vi "start.vi"(8 "error in (no error)":errorcluster, 10 "model":refnum<class "Model.lvclass">, 11 "StandbyState in":refnum<class "StandbyState.lvclass">) -> (0 "error out":errorcluster, 2 "model 2":refnum<class "Model.lvclass">, 3 "StandbyState out":refnum<class "StandbyState.lvclass">)   [LabVIEW 2013, in "StandbyState.lvclass"]
uses:
  StandbyState.lvclass
  Model/Model/Model.lvclass
  Typedefs/StateSelector.ctl
  Typedefs/AITDTTypedefs.lvlib
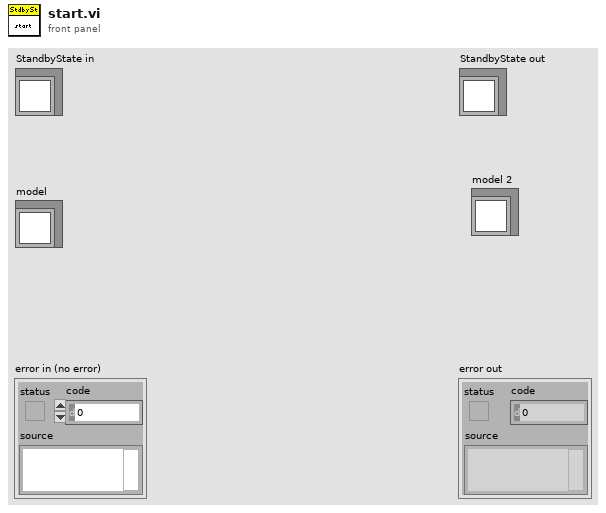
[diagram p1: front panel]
types:
  T1 = typedef "AITDTTypedefs.lvlib/StateSelector.ctl" = enum16{"AwaitingSetpointAcknowledgmentState", "EndingCycleState", "FaultState", "OffState", "PausingState", "RequestingNewSetpointState", "SamplingState", "SettlingState", "SoakingState", "StabilizingState", "StandbyState", "StoppedState", "TransitioningTemperatureState"}
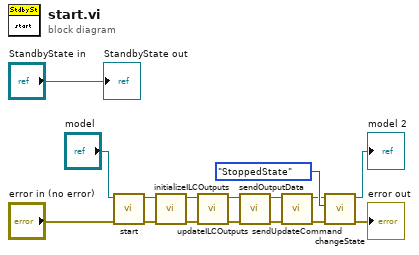
[diagram p0: block diagram]
diagram:
  n1 = call "start.vi"("error in (no error)"="error in (no error)", "Model in"="model") -> ("error out"=w9:errorcluster, "Model out"=w10:refnum<class "Model.lvclass">)  [unwired: 8 in]
  n2 = call "initializeILCOutputs.vi"("error in (no error)"=w9, "Model in"=w10) -> ("error out"=w1:errorcluster, "Model out"=w2:refnum<class "Model.lvclass">)  [unwired: 8 in]
  n3 = call "updateILCOutputs.vi"("error in (no error)"=w1, "Model in"=w2) -> ("error out"=w7:errorcluster, "Model out"=w8:refnum<class "Model.lvclass">)  [unwired: 8 in]
  n4 = call "sendOutputData.vi"("error in (no error)"=w7, "Model in"=w8) -> ("error out"=w3:errorcluster, "Model out"=w4:refnum<class "Model.lvclass">)  [unwired: 8 in]
  n5 = call "sendUpdateCommand.vi"("error in (no error)"=w3, "Model in"=w4) -> ("error out"=w5:errorcluster, "Model out"=w6:refnum<class "Model.lvclass">)  [unwired: 8 in]
  n6 = call "changeState.vi"("error in (no error)"=w5, "State:"=StateSelector."StoppedState", "Model in"=w6) -> ("error out"=→"error out":errorcluster, "Model out"=→"model 2":refnum<class "Model.lvclass">)  [unwired: 7 in]
  "StandbyState out" <- "StandbyState in"
